vi "HEWH RLT PRAT.vi"() -> ()   [LabVIEW 2016] (continued)
        w1531 = 42 items=["No error", "Argument error", "Memory is full", "Out of zone", "End of file", "File already open", "Generic file I/O error", "File not found", "File permission error", "Disk is full", "Duplicate path", "Too many files open", "System feature not enabled", "Resource file not found", "Cannot add resource", "Resource not found", "Image not found", "Image memory error", "Pen does not exist", "Config type invalid", "Config token not found", "Config parse error", "Config memory error", "Bad external code format", "Bad external code offset", "External code not present", "Null window", "Destroy window error", "Null menu", "Print aborted", "Bad print record", "Print driver error", "Windows error during printing", "Memory error during printing", "Print dialog error", "Generic print error", "Invalid device refnum", "Device not found", "Device parameter error", "Device unit error", "Cannot open device", "Device call aborted", "Generic error", "Cancelled by user", "Object ID too low", "Object ID too high", "Object not in heap", "Unknown heap", "Unknown object (invalid DefProc)", "Unknown object (DefProc not in table)", "Message out of range", "Invalid (null) method", "Unknown message", "Manager call not supported", "Bad address", "Network operation in progress", "Network operation timed out", "Connection is busy", "Network attribute not supported", "Network error", "Address in use", "System out of memory", "Connection aborted", "Connection refused", "Not connected", "Already connected", "Connection closed", "Initialization error (interapplication manager)", "Bad occurrence", "Wait on unbound occurrence handler", "Occurrence queue overflow", "Datalog type conflict", "Unused", "Unrecognized type (interapplication manager)", "Memory corrupt", "Failed to make temporary DLL", "Old CIN version", "Drag socket not found", "Failed to load drop-object", "Failed to register OLE object", "Failed to release OLE object", "Format specifier type mismatch", "Unknown format specifier", "Too few format specifiers", "Too many format specifiers", "Scan failed", "Newer CIN version", "Error converting to variant", "Runtime menu error", "Password tampered", "Variant attribute not found", "Incompatible variant data type", "Event data is not available", "Event Store is not present", "Occurrence is not found", "Event Queue is not created", "Event info is not available", "Refnum passed is NULL", "Error retrieving Class GUID", "Error retrieving CoClass GUID", "Error retrieving TypeLib GUID.", "Bad built application magic bytes.", "Specific driver is different from the specific driver associated with the Logical Name.", "There is no session opened to the class driver.", "Max Error", "MAX - Error with config objects", "MAX - Error loading configuration", "MAX - Group not supported"]
        # "Current State"
        # "Handle mistyped state name (developer tool)"
        n704 = Format Into String(format string="Software Exception: Unhandled State \"%s\"." ("message"), error in=w1527, w1523) -> (resulting string=w1530:string, error out=w1529:errorcluster)  [unwired: 1 in]
        n705 = call <vilib>:"Error Cluster From Error Code.vi"("show call chain? (False)"=TRUE, "error in (no error)"=w1529, "error message (\"\")"=w1530, "error code (0)"=w1531) -> ("error out"=w1528:errorcluster)  [unwired: 5 in]
        n706 = call <vilib>:"Add State(s) to Queue__jki_lib_state_machine.vi"("State(s) in (\"\")"=w1526) -> ("States Out"=w1525:string)  [unwired: 14 in]
      }
      frame "Error Handler" {
        # "Unhandled Error -- Display it"
        # "Clear error"
        n707 = call <vilib>:"General Error Handler.vi"("error in (no error)"=w1534) -> ()  [unwired: 10 in, 5 out]
        n708 = call <vilib>:"Add State(s) to Queue__jki_lib_state_machine.vi"("State(s) in Front (\"\")"="/* Post Error States", "State(s) in (\"\")"=w1538) -> ("States Out"=w1537:string)  [unwired: 13 in]
      }
      frame "Exit" {
        n709 = flat-sequence {
          tunnel: w1543 -> [w1548]
          tunnel: [w1548] -> w1539
          tunnel: [w1551] -> w1541
          tunnel: w1539 -> [w1552]
          tunnel: [w1554] -> w1542
          tunnel: w1541 -> [w1554]
          tunnel: [TRUE] -> w1540
          frame #0 {
            n710 = local read "Start Draw"() -> (w1547:bool)
            n711 = case shown="True" w1547 {
              frame False {
              }
              frame True {
                n712 = while {
                  stop <- w1550 stop-if-true
                  n713 = local read "Draw Complete"() -> (w1550:bool)
                  n714 = Wait Until Next ms Multiple(millisecond multiple=u32 100) -> ()  [unwired: 1 out]
                }
              }
            }
          }
          frame #1 {
            n715 = call "HEWH RLT Release Notifier References.vi"("error in (no error)"=w1552) -> ("error out"=w1551:errorcluster)  [unwired: 10 in]
          }
          frame #2 {
          }
        }
        n716 = call <vilib>:"Add State(s) to Queue__jki_lib_state_machine.vi"("State(s) in (\"\")"=w1546) -> ("States Out"=w1545:string)  [unwired: 14 in]
        "DAQ Finished" <- w1540
      }
      frame "---------- Setup ----------" {
        n717 = call <vilib>:"Add State(s) to Queue__jki_lib_state_machine.vi"("State(s) in (\"\")"=w1558) -> ("States Out"=w1557:string)  [unwired: 14 in]
      }
      frame "Data: Initialize" {
        n718 = while {
          tunnel: ["Test Fixture Hardware"] -> w1570
          tunnel: [w1612] -> w1586
          tunnel: [w1611] -> w1585
          tunnel: [w1610] -> w1584
          tunnel: [w1609] -> w1583
          tunnel: [w1608] -> w1582
          tunnel: [w1607] -> w1581
          tunnel: ["Core HEWH Data Input A"] -> w1573
          tunnel: ["Core HEWH Data Input B"] -> w1580
          tunnel: ["Core HEWH Data Input C"] -> w1579
          tunnel: ["Core HEWH Data Input D"] -> w1578
          tunnel: ["File Locations A"] -> w1577
          tunnel: ["File Locations B"] -> w1576
          tunnel: ["File Locations C"] -> w1575
          tunnel: ["File Locations D"] -> w1574
          tunnel: [w1596] -> w1568
          tunnel: [w1595] -> w1567
          tunnel: [w1594] -> w1566
          tunnel: [w1593] -> w1565
          tunnel: [w1592] -> w1564
          tunnel: [w1591] -> w1563
          tunnel: [w1590] -> w1560
          tunnel: [w1589] -> w1559
          stop <- w1606 stop-if-true
          w1592 = dbl[][] []  # Plot Array C
          w1591 = dbl[][] []  # Plot Array D
          w1593 = dbl[][] []  # Plot Array B
          w1594 = dbl[][] []  # Plot Array A
          w1608 = string[][] []  # D Data Array
          w1609 = string[][] []  # C Data Array
          w1610 = string[][] []  # B Data Array
          w1611 = string[][] []  # A Data Array
          w1612 = string[][] []  # Save Data
          n719 = local read "Init Complete"() -> (w1606:bool)
          n720 = local read "LV Program"() -> (w1596:T24)
          n721 = Wait Until Next ms Multiple(millisecond multiple=u32 100) -> ()  [unwired: 1 out]
          n722 = local read "Analog Channel-List"() -> (w1589:string)
          n723 = local read "RLT Station Channels"() -> (w1607:T46)
          n724 = local read "Scan Rate (Seconds)"() -> (w1590:T10)
          n725 = local read "Power Analyzer"() -> (w1595:T11)
        }
        n726 = call <vilib>:"Add State(s) to Queue__jki_lib_state_machine.vi"("State(s) in (\"\")"=w1588) -> ("States Out"=w1587:string)  [unwired: 14 in]
        n727 = Bundle("Test Fixture Hardware"=w1570, "Save Data"=w1586, "A Data Array"=w1585, "B Data Array"=w1584, "C Data Array"=w1583, "D Data Array"=w1582, "RLT Station Channels"=w1581, "Core HEWH Data Input A"=w1573, "Core HEWH Data Input B"=w1580, "Core HEWH Data Input C"=w1579, "Core HEWH Data Input D"=w1578, "File Locations A"=w1577, "File Locations B"=w1576, "File Locations C"=w1575, "File Locations D"=w1574, "Plot Array A"=w1566, "Plot Array B"=w1565, "Plot Array C"=w1564, "Plot Array D"=w1563, "Scan Rate (Seconds)"=w1560) -> (w1571:T80)  [unwired: 1 in]
        n728 = Unbundle By Name(w1570) -> ("Analog Data.Yokogawa.MW100"=→"MW100":refnum<visa-resource-name>, "Power.Yokogawa.WT210.Power VISA Yokogawa WT210"=→"Yokogawa WT210":refnum<visa-resource-name>)
        n729 = Bundle By Name(cluster=w1571, "Core HEWH Data Input A.HEWH Specific DAQ.Power Analyzer"=w1567, "Core HEWH Data Input B.HEWH Specific DAQ.Power Analyzer"=w1567, "Core HEWH Data Input C.HEWH Specific DAQ.Power Analyzer"=w1567, "Core HEWH Data Input D.HEWH Specific DAQ.Power Analyzer"=w1567, "Core HEWH Data Input A.LV Program"=w1568, "Core HEWH Data Input B.LV Program"=w1568, "Core HEWH Data Input C.LV Program"=w1568, "Core HEWH Data Input D.LV Program"=w1568, "Test Fixture Hardware.Analog Data.Agilent.TC Channels-List"=w1559) -> (w1572:T80)
      }
      frame "Initialize Equipment" {
        w1624 = 0 ("Core HEWH Data Input A.Draw Count")
        # "The Initialize Equipment only requires VISA connections. We use\na single MW100, WT Series, and 34972A"
        n730 = Unbundle By Name(w1632) -> ("Test Fixture Hardware"=w1633:T47, "Core HEWH Data Input A"=w1634:T12, "Test Fixture Hardware.Gas Meter COM Ports.Gas Meter 1"=w1619:refnum<visa-resource-name>)
        n731 = local read "Use Agilent?"() -> (w1623:bool)
        n732 = call "HEWH Initialize Equipmet.vi"("Refnum in"=w1625, "Use Agilent?"=w1623, "Error In"=w1626, "Pressurize Tank"="Pressurize Tank?", "Core HEWH Data"=w1634, "Test Fixture Hardware"=w1633) -> ("Error Out"=w1621:errorcluster)  [unwired: 4 in, 1 out]
        n733 = call "FMA1600A General Setup.vi"("baud rate (19200)"=u32 19200 ("baud rate (9600)"), "Unit ID"="A", "error in (no error)"=w1621, "Set STP Register"=FALSE, "VISA Refnum in"=w1619) -> ("error out"=w1617:errorcluster, "VISA Refnum out"=w1614:refnum<visa-resource-name>)  [unwired: 4 in, 1 out]
        n734 = call <vilib>:"Add State(s) to Queue__jki_lib_state_machine.vi"("State(s) in (\"\")"=w1637) -> ("States Out"=w1636:string)  [unwired: 14 in]
        n735 = Bundle By Name(cluster=w1632, "Core HEWH Data Input A.Station ID"=Station_ID_Selector."A", "Core HEWH Data Input B.Station ID"=Station_ID_Selector."B", "Core HEWH Data Input C.Station ID"=Station_ID_Selector."C", "Core HEWH Data Input D.Station ID"=Station_ID_Selector."D", "Core HEWH Data Input A.Draw Count"=w1624, "Core HEWH Data Input B.Draw Count"=w1624, "Core HEWH Data Input C.Draw Count"=w1624, "Core HEWH Data Input D.Draw Count"=w1624, "Test Fixture Hardware.Gas Meter COM Ports.Gas Meter 1"=w1614) -> (w1631:T80)
        n736 = call <vilib>:"Clear Errors.vi"("error in (no error)"=w1617, "specific error code to clear (0: all)"=0) -> ("error out"=w1616:errorcluster)  [unwired: 4 in, 1 out]
      }
      frame "Get Software Version A" {
        w1645 = "." ("string")
        w1652 = GEA2_Commands."RQST_Software_Version" ("GEA2 Commands and Requests")
        n737 = Unbundle By Name(w1643) -> ("Board ID"=→"Board ID A":string, "GEA2 Reference Out"=w1642:refnum<k24>, "GEA2 Event Registration"=w1641:refnum<event-registration>)
        n738 = call "HEWH_DSM_CMD.vi"("GEA2 Commands and Requests"=w1652) -> ("Input Data"=w1651:T74)  [unwired: 8 in, 1 out]
        n739 = call "GEA2 Send and Receive Message.vi"("GEA2 Reference In"=w1642, "Input Data"=w1651, "GEA2 Event Registration"=w1641, "Error In"=w1640) -> ("Converted Data Out"=w1653:T81, "Error Out"=w1639:errorcluster)  [unwired: 6 in, 4 out]
        n740 = call "GEA2 Message Decoder.vi"("GEA2 Commands and Requests"=w1652, "Coverted Data Out"=w1653) -> ("GEA Information Out"=w1650:T57)  [unwired: 9 in]
        n741 = Unbundle By Name(w1650) -> ("Software Version.Critical Major SW Version"=w1649:string, "Software Version.Critical Minor SW Version"=w1648:string, "Software Version.Major SW Version"=w1647:string, "Software Version.Minor SW Version"=w1646:string)
        n742 = Concatenate Strings(w1649, w1645, w1648, w1645, w1647, w1645, w1646) -> (→"Software Version A":string)
        n743 = call <vilib>:"Add State(s) to Queue__jki_lib_state_machine.vi"("State(s) in (\"\")"=w1656) -> ("States Out"=w1655:string)  [unwired: 14 in]
      }
      frame "Get Software Version B" {
        w1664 = "." ("string")
        w1671 = GEA2_Commands."RQST_Software_Version" ("GEA2 Commands and Requests")
        n744 = Unbundle By Name(w1662) -> ("Board ID"=→"Board ID B":string, "GEA2 Reference Out"=w1661:refnum<k24>, "GEA2 Event Registration"=w1660:refnum<event-registration>)
        n745 = call "HEWH_DSM_CMD.vi"("GEA2 Commands and Requests"=w1671) -> ("Input Data"=w1670:T74)  [unwired: 8 in, 1 out]
        n746 = call "GEA2 Send and Receive Message.vi"("GEA2 Reference In"=w1661, "Input Data"=w1670, "GEA2 Event Registration"=w1660, "Error In"=w1659) -> ("Converted Data Out"=w1672:T81, "Error Out"=w1658:errorcluster)  [unwired: 6 in, 4 out]
        n747 = call "GEA2 Message Decoder.vi"("GEA2 Commands and Requests"=w1671, "Coverted Data Out"=w1672) -> ("GEA Information Out"=w1669:T57)  [unwired: 9 in]
        n748 = Unbundle By Name(w1669) -> ("Software Version.Critical Major SW Version"=w1668:string, "Software Version.Critical Minor SW Version"=w1667:string, "Software Version.Major SW Version"=w1666:string, "Software Version.Minor SW Version"=w1665:string)
        n749 = Concatenate Strings(w1668, w1664, w1667, w1664, w1666, w1664, w1665) -> (→"Software Version B":string)
        n750 = call <vilib>:"Add State(s) to Queue__jki_lib_state_machine.vi"("State(s) in (\"\")"=w1675) -> ("States Out"=w1674:string)  [unwired: 14 in]
      }
      frame "Get Software Version C" {
        w1683 = "." ("string")
        w1690 = GEA2_Commands."RQST_Software_Version" ("GEA2 Commands and Requests")
        n751 = Unbundle By Name(w1681) -> ("Board ID"=→"Board ID C":string, "GEA2 Reference Out"=w1680:refnum<k24>, "GEA2 Event Registration"=w1679:refnum<event-registration>)
        n752 = call "HEWH_DSM_CMD.vi"("GEA2 Commands and Requests"=w1690) -> ("Input Data"=w1689:T74)  [unwired: 8 in, 1 out]
        n753 = call "GEA2 Send and Receive Message.vi"("GEA2 Reference In"=w1680, "Input Data"=w1689, "GEA2 Event Registration"=w1679, "Error In"=w1678) -> ("Converted Data Out"=w1691:T81, "Error Out"=w1677:errorcluster)  [unwired: 6 in, 4 out]
        n754 = call "GEA2 Message Decoder.vi"("GEA2 Commands and Requests"=w1690, "Coverted Data Out"=w1691) -> ("GEA Information Out"=w1688:T57)  [unwired: 9 in]
        n755 = Unbundle By Name(w1688) -> ("Software Version.Critical Major SW Version"=w1687:string, "Software Version.Critical Minor SW Version"=w1686:string, "Software Version.Major SW Version"=w1685:string, "Software Version.Minor SW Version"=w1684:string)
        n756 = Concatenate Strings(w1687, w1683, w1686, w1683, w1685, w1683, w1684) -> (→"Software Version C":string)
        n757 = call <vilib>:"Add State(s) to Queue__jki_lib_state_machine.vi"("State(s) in (\"\")"=w1694) -> ("States Out"=w1693:string)  [unwired: 14 in]
      }
      frame "Get Software Version D" {
        w1702 = "." ("string")
        w1709 = GEA2_Commands."RQST_Software_Version" ("GEA2 Commands and Requests")
        n758 = Unbundle By Name(w1700) -> ("Board ID"=→"Board ID D":string, "GEA2 Reference Out"=w1699:refnum<k24>, "GEA2 Event Registration"=w1698:refnum<event-registration>)
        n759 = call "HEWH_DSM_CMD.vi"("GEA2 Commands and Requests"=w1709) -> ("Input Data"=w1708:T74)  [unwired: 8 in, 1 out]
        n760 = call "GEA2 Send and Receive Message.vi"("GEA2 Reference In"=w1699, "Input Data"=w1708, "GEA2 Event Registration"=w1698, "Error In"=w1697) -> ("Converted Data Out"=w1710:T81, "Error Out"=w1696:errorcluster)  [unwired: 6 in, 4 out]
        n761 = call "GEA2 Message Decoder.vi"("GEA2 Commands and Requests"=w1709, "Coverted Data Out"=w1710) -> ("GEA Information Out"=w1707:T57)  [unwired: 9 in]
        n762 = Unbundle By Name(w1707) -> ("Software Version.Critical Major SW Version"=w1706:string, "Software Version.Critical Minor SW Version"=w1705:string, "Software Version.Major SW Version"=w1704:string, "Software Version.Minor SW Version"=w1703:string)
        n763 = Concatenate Strings(w1706, w1702, w1705, w1702, w1704, w1702, w1703) -> (→"Software Version D":string)
        n764 = call <vilib>:"Add State(s) to Queue__jki_lib_state_machine.vi"("State(s) in (\"\")"=w1713) -> ("States Out"=w1712:string)  [unwired: 14 in]
      }
      frame "Update File Locations" {
        n765 = flat-sequence {
          tunnel: w1715 -> [w1729]
          tunnel: w1720 -> [w1728]
          tunnel: w1719 -> [w1727]
          tunnel: w1718 -> [w1726]
          tunnel: w1717 -> [w1725]
          tunnel: [w1724] -> w1716
          tunnel: w1716 -> [w1731]
          tunnel: [w1731] -> w1714
          frame #0 {
            n766 = Bundle By Name(cluster=w1729, "File Locations A"=w1728, "File Locations B"=w1727, "File Locations C"=w1726, "File Locations D"=w1725) -> (w1724:T80)
          }
          frame #1 {
            n767 = Unbundle By Name(w1731) -> ("Core HEWH Data Input A"=w1735:T12, "Core HEWH Data Input B"=w1734:T12, "Core HEWH Data Input C"=w1733:T12, "Core HEWH Data Input D"=w1732:T12, "Scan Rate (Seconds)"=→"Scan Rate (Default)":T10)
            n768 = local write "Core HEWH Data Input A"(w1735) -> ()
            n769 = local write "Core HEWH Data Input B"(w1734) -> ()
            n770 = local write "Core HEWH Data Input C"(w1733) -> ()
            n771 = local write "Core HEWH Data Input D"(w1732) -> ()
          }
          frame #2 {
            "Start Draw Loop" <- TRUE ("Init Complete")
          }
        }
        n772 = call <vilib>:"Add State(s) to Queue__jki_lib_state_machine.vi"("State(s) in (\"\")"=w1723) -> ("States Out"=w1722:string)  [unwired: 14 in]
      }
      frame "Load Configuration" {
        n773 = Unbundle By Name(w1742) -> ("Core HEWH Data Input A.LV Program"=w1746:T24, "File Locations A"=w1745:T2)
        n774 = call "Save File DOE File Setup.vi"("Filepath In"=w1745, "Washer Controls In"=T75 {"Test Fixture Hardware"={"Power "={"Yokogawa"={"WT210"={"Sample Rate (1: 0.25s)"=1, "A Range (12: 20A)"=12, "V Range (6: 600V)"=4, "Power VISA Yokogawa WT210"="WT210"}, "WT500"={"Power VISA Yokogawa WT500"="WT500", "V Range (8: 1000V)"=0, "I Range (7: 40A)"=0, "Update Rate (3: 500ms)"=2}, "WT310_2"={"Sample Rate (1: 0.25s)"=1, "A Range (12: 20A)"=11, "V Range (6: 600V)"=4, "Power VISA Yokogawa WT310_2"=""}, "WT310_3"={"Sample Rate (1: 0.25s)"=1, "A Range (12: 20A)"=11, "V Range (6: 600V)"=4, "Power VISA Yokogawa WT310_3"=""}}, "Aplus"={"Aplus IP Address"="192.168.1.101", "Remote Port"=502, "Instrument"="APLUS", "Instr Driver Revision"="1.03.0053"}, "Power Limits"={"Crest Factor"={"Upper Limit"=1.49, "Lower Limit"=1.34}, "Harmonic Content"={"Uthd"=2.0}, "Voltage"={"% Error"=2.0}, "Stability"={"<1 Watt "={"Wattage"=1.0, "Slope (mW/H)"=10.0}, ">1 Watt"={"1%Power/Hour"=1.0}}}, "Nominal Voltage"=120, "Time Limit (s)"=10800.0, "Power Variation Limit (%)"=50.0, "Power Supply"={"Chroma 61605"="CHROMA", "Use Chroma?"=FALSE}}, "Weight Scale"={"Com Options"={"IND560Scale VISA"="IND560", "IP Address"="192.168.1.50", "Remote Port"=502, "Setra Scale VISA"="COM3", "GSE 350"="GSE350"}, "Select Scale"=""}, "Flow Rates"={"Laurel Cold IP Address"="", "Laurel Hot IP Address"="34972A_2", "Hot Water Laurel VISA"="LaurelMeter_Hot", "Cold Water Laurel VISA"="LaurelMeter_Cold", "Remote Port"=0, "Laurel Communication Type"="", "Meters To Collect (Hot Cold)"="", "HOT Laurel Reference"=refnum, "COLD Laurel Reference"=refnum}, "Analog Data"={"Agilent"={"Agilent 34972_1"="34972A_1", "Agilent 34972_2"="34972A_2", "Agilent 34972_3"="34972A_3", "Agilent 34972_4"="34972A_4", "Agilent 34972_5"="34972A_5", "Agilent 34972_6"="34972A_6", "Agilent Gain"=0.0, "TC Type (K,J,T)"="", "Instrument IDN?"="", "TC Channels-List"="", "Analog Channels-List"="", "Agilent Cluster Array"=[], "TC Channels-List 2"="", "Analog Channels-List 2"=""}, "Yokogawa"={"MW100"="MW100", "Intellifaucet"=FALSE}, "Select Analog"="", "TC Coefficients"={"TC Coefficients 1"=[], "TC Coefficients 2"=[], "TC Coefficients 3"=[], "TC Coefficients 4"=[], "TC Coefficients 5"=[], "TC Coefficients 6"=[], "TC Coefficients 7"=[]}, "NI Tasks (Dryer DOE)"=["TC Temps-Module 1", "TC Temps-Module 2", "TC Temps-Module 3", "TC Temps-Module 4", "TC Temps-Module 5", "Gas and Temp-Module 6", "AC_DC Events-Module 7"], "Laurel Analog"={"Laurel IP (Water Temp)"="", "Laurel IP (Pressure)"=""}}, "ITHX-Temp Humidity"={"IP Address 1"="", "Remote Port"=0, "IP Address 2"="", "IP Address 3"=""}, "Gas Meter COM Ports"={"Gas Meter 1"="COM3", "Gas Meter 2"="COM4", "Gas Meter 3"="COM5", "Gas Meter 4"="COM6", "Gas Meter 5"="COM7", "Gas Meter 6"="COM8"}, "Barometric Pressure"={"HEISE 901A"="HEISE", "Use Barometer?"=FALSE}}, "GEA2"={"Address"=35, "Source"=228, "Viper/Hawk"=0}, "DOE Capacity Measurments"={"Weight 1"=35.0, "Model Number 1"="", "Temp 1"=0.0, "Serial Number 1"="", "Lab Number 1"="", "Lab Number 2"="", "Serial Number 2"="", "Temp 2"=0.0, "Model Number 2"="", "Weight 2"=0.0, "Lab Number 3"="", "Serial Number 3"="", "Temp 3"=0.0, "Model Number 3"="", "Weight 3"=0.0, "Lab Number 4"="", "Serial Number 4"="", "Temp 4"=0.0, "Model Number 4"="", "Weight 4"=0.0, "Capacity Measurment Output String"=[]}, "Initialize.Washer In"={"Appliance Details"={"FileVersionInfo"={"FileVersion"="", "ProductName"="", "InternalName"="", "CompanyName"="", "LegalCopyright"="", "FileDescription"=""}, "Dishwasher Info"={"Open Cup Weight (gm):"=0.0, "Auto Cup Weight (gm):"=0.0, "Detergent-Dish:"="", "Inlet Temperature-Dish:"="", "Cycle Mode-Dish:"="", "Unit Control-Dish:"="", "Manufacturer-Dish:"=""}, "Washer Info"={"Hot Water Temperature (Fahrenheit):"="", "Cold Water Temperature (Fahrenheit):"="", "Capacity (cu.ft):"=0.0, "Initial Cloth Weight:"=0.0, "Cloth Lot:"=60, "Model Family:"="", "Program Name:"="", "Cycle Selection:"="", "Wash Temperature:"="", "Rinse Temperature:"="", "Load Size:"=""}, "File Name Output Array"=[], "Calibration Output Array"=[], "Appliance Common"={"Engineer:"="", "Model Number:"="", "Serial Number:"="", "Comments:"="", "Station ID:"="", "Technician:"="", "TR Number:"="", "Lab ID:"="", "Voltage:"="", "Water Pressure (PSI):"="", "Test Date:"="", "Computer Name:"="", "IP Address:"="", "Ambient RH:"="", "Frequency:"="", "Build:"="", "Filename:"="", "Test Type:"="", "Load Run #:"=17, "Ambient Temperature (F):"="", "File Path:"=path "", "Cycles Per Year"=0}, "Water Heater"={"Heating Mode:"=""}, "Dryer"={"Heat Setting:"="", "Washer Water Temperature (60 ± 5°F):"=7, "Water Hardness (PPM):"=7, "Dryness Setting:"="", "Dryer Type:"="", "Exhaust:"="", "Drying Cycle:"="", "Load Type:"="", "Nominal Load Weight"="", "Dryer Initial IMC Data"={"Measured IMC (lbs)"=100.0, "Actual Initial RMC (%)"=7.0, "RMC (Desired %)"=5.0, "Bone Dry Wt(lbs)"=60.0, "Tolerance(%)"=0.0, "Actual Final RMC (%)"=0.0, "CEF (lbf/kWh)"=0.0, "Minimum Weight (lbf)"=0.0, "Average Weight (lbf)"=0.0, "Maximum Weight (lbf)"=0.0, "Measured IMC In Range?"=FALSE, "Moisture Reduction Factor"=55.5, "Field Use Factor"=1.04, "Empty Dryer Cold Weigth"=0.0, "Energy Standard"=enum."D2-Automatic Dryer", "Weight Cloth (lbs)"=0.0, "Relative Moisture Content (%)"=0.0, "Relative Moisture Content - Avg (%)"=0.0}}}, "Display Data (RLT)"={"Status Color"=0, "Serial Number Display"="", "Cycle Count Display"=0, "Station Label Display"="", "Current Run Start Time Display"=0.0, "Board ID Display"="", "RPM Display"=0, "Current Display"=0.0, "Current Path Display"=path "", "Saving Display"=FALSE, "Unit Type Display"=enum."", "Total Time On Display"=0.0, "UI Button"=FALSE}}}, "error in (no error)"=w1748, "Config State"=Save_File_DOE_Configuration_State."Load Config", "LV Program"=w1746) -> ("Washer Controls Out"=w1743:T75, "Filepath Out"=w1738:T2, "error out"=w1747:errorcluster)  [unwired: 12 in]
        n775 = Unbundle By Name(w1743) -> ("Test Fixture Hardware.ITHX-Temp Humidity.IP Address 1"=w1741:string, "Test Fixture Hardware.Flow Rates.Laurel Hot IP Address"=w1739:string)
        "ITHX-Temp Humidity" <- w1741
        "Laurel Hot IP Address" <- w1739
        n776 = call <vilib>:"Add State(s) to Queue__jki_lib_state_machine.vi"("State(s) in (\"\")"=w1751) -> ("States Out"=w1750:string)  [unwired: 14 in]
        n777 = Bundle By Name(cluster=w1742, "Test Fixture Hardware.ITHX-Temp Humidity.Remote Port"=u16 2000, "Test Fixture Hardware.ITHX-Temp Humidity.IP Address 1"=w1741, "Test Fixture Hardware.Flow Rates.Laurel Hot IP Address"=w1739, "File Locations A"=w1738, "File Locations B"=w1738, "File Locations C"=w1738, "File Locations D"=w1738) -> (w1737:T80)
      }
      frame "Init Hot Laurel" {
        n778 = Unbundle By Name(w1755) -> ("Test Fixture Hardware.Flow Rates.Laurel Hot IP Address"=w1752:string)
        n779 = Equal?(x=w1752, y="") -> (x = y?=w1753:bool)
        n780 = case shown="False" w1753 {
          tunnel: w1752 -> [_ w1763]
          tunnel: w1757 -> [w1760 w1762]
          tunnel: [w1760 w1765] -> w1756
          frame True {
          }
          frame False {
            n781 = call "Emerson 5700 Basic Tester.vi"("Error In"=w1762, "Remote IP Address"=w1763) -> ("Error Out"=w1761:errorcluster)  [unwired: 8 in, 1 out]
            n782 = case shown="Error" w1761 {
              selector: w1761 -> [w1774 _]
              tunnel: [w1769 w1781] -> w1765
              tunnel: w1763 -> [w1767 w1779]
              tunnel: [TRUE ("Use Emerson 5700") FALSE ("Use Emerson 5700")] -> w1764
              frame No Error {
                w1768 = T82 4 items=["Start/Stop Inventory 1"=367, "Start/Stop Inventory 2"=368, "Start/Stop all Totalizers and Inventories"=2, "Reset all Totalizers"=3, "Reset all Inventories"=4, "Reset Totalizer 1"=56, "Reset Totalizer 2"=57] ("Reset all Totalizers. 2")
                w1772 = T82 3 items=["Start/Stop Inventory 1"=367, "Start/Stop Inventory 2"=368, "Start/Stop all Totalizers and Inventories"=2, "Reset all Totalizers"=3, "Reset all Inventories"=4, "Reset Totalizer 1"=56, "Reset Totalizer 2"=57] ("Reset all Totalizers. 2")
                n783 = property on="Reset Inventory" class="Bool"("DisabledEnum"=T67."Enabled" ("Disabled")) -> ()  [unwired: 2 in, 2 out]
                n784 = call "Emerson 5700 Reset Totalizers.vi"("Reset all Totalizers. 2"=w1772, "Error In"=w1774, "Coil"=TRUE, "address"=w1767) -> ("Error Out"=w1770:errorcluster)  [unwired: 7 in]
                n785 = call "Emerson 5700 Reset Totalizers.vi"("Reset all Totalizers. 2"=w1768, "Error In"=w1770, "Coil"=TRUE, "address"=w1767) -> ("Error Out"=w1769:errorcluster)  [unwired: 7 in]
              }
              frame Error {
                n786 = for {
                  N: 2 -> [_]
                  tunnel: w1779 -> [w1785]
                  tunnel: errorcluster {"status"=FALSE, "code"=0, "source"=""} ("Error Out") -> [w1784]
                  tunnel: [w1783] -> w1781
                  n787 = First Call?() -> (First Call?: T/F=w1787:bool)
                  n788 = call "Laurel Data GET Top Level.vi"("Laurel IP Address"=w1785, "Laurel Serial Commands"=T79 "*1C1", "First Call?"=w1787, "error in (no error)"=w1784, "Laurel Communication Type"="TCP") -> ("error out"=w1783:errorcluster)  [unwired: 5 in, 5 out]
                }
                n789 = property on="Reset Inventory" class="Bool"("DisabledEnum"=T67."Disabled and Grayed Out" ("Disabled")) -> ()  [unwired: 2 in, 2 out]
              }
            }
            "Use Emerson 5700" <- w1764
          }
        }
        n790 = call <vilib>:"Add State(s) to Queue__jki_lib_state_machine.vi"("State(s) in (\"\")"=w1759) -> ("States Out"=w1758:string)  [unwired: 14 in]
      }
      frame "Shutdown Equipment" {
        n791 = Unbundle By Name(w1797) -> ("Test Fixture Hardware"=w1796:T47, "Core HEWH Data Input A"=w1795:T12, "Test Fixture Hardware.Gas Meter COM Ports.Gas Meter 1"=w1789:refnum<visa-resource-name>)
        n792 = local read "Pressurize Tank?"() -> (w1794:bool)
        n793 = local read "Get Gas Data"() -> (w1788:bool)
        n794 = call "HEWH Close Equipmet.vi"("Refnum in"=w1792, "Pressurize Tank"=w1794, "Error In"=w1793, "Core HEWH Data"=w1795, "Test Fixture Hardware In"=w1796) -> ("Error Out"=w1791:errorcluster)  [unwired: 5 in, 1 out]
        n795 = case shown="True" w1788 {
          tunnel: w1791 -> [w1800 w1803]
          tunnel: [w1800 w1802] -> w1790
          tunnel: w1789 -> [_ w1801]
          frame False {
          }
          frame True {
            n796 = call "FMA1600A Close.vi"("error in (no error)"=w1803, "VISA Refnum in"=w1801) -> ("error out"=w1802:errorcluster)  [unwired: 9 in]
          }
        }
        n797 = call <vilib>:"Add State(s) to Queue__jki_lib_state_machine.vi"("State(s) in (\"\")"=w1799) -> ("States Out"=w1798:string)  [unwired: 14 in]
      }
      frame "---------- Data ----------" {
        n798 = call <vilib>:"Add State(s) to Queue__jki_lib_state_machine.vi"("State(s) in (\"\")"=w1807) -> ("States Out"=w1806:string)  [unwired: 14 in]
      }
      frame "Data: Get Time" {
        w1808 = i16 2 ("precision (6)")
        w1809 = TRUE ("Add Software Elapsed Time")
        w1835 = string[][] [] ("A Data Array")
        # "allows reset after purge"
        # "Reset Array"
        n799 = call "UTILITY Elapsed Time.vi"("error in (no error)"=w1812, "Reset Timer"="Reset Timer (Main)") -> ("error out"=w1811:errorcluster, "Main Loop Rate"=→"DAQ Loop Rate":dbl, "Elapsed Time"=w1810:dbl)  [unwired: 5 in, 2 out]
        "Software Elapsed Time" <- w1810
        n800 = Bundle By Name(cluster=w1833, "A Data Array"=w1835, "B Data Array"=w1835, "C Data Array"=w1835, "D Data Array"=w1835) -> (w1834:T80)
        n801 = local read "A Timer"() -> (w1824:dbl)
        n802 = local read "B Timer"() -> (w1820:dbl)
        n803 = call "UTILITY Elapsed Time General Info.vi"("precision (6)"=w1808, "Add Software Elapsed Time"=w1809, "Error In"=w1811, "Software Elapsed Time"=w1810, "Elapsed Time (sec)"=w1824) -> ("Error Out"=w1822:errorcluster, "Total Array"=w1823:string[][])  [unwired: 2 in, 3 out]
        n804 = local read "C Timer"() -> (w1815:dbl)
        n805 = call "UTILITY Elapsed Time General Info.vi"("precision (6)"=w1808, "Add Software Elapsed Time"=w1809, "Error In"=w1822, "Software Elapsed Time"=w1810, "Elapsed Time (sec)"=w1820) -> ("Error Out"=w1819:errorcluster, "Total Array"=w1821:string[][])  [unwired: 2 in, 3 out]
        n806 = call "UTILITY Elapsed Time General Info.vi"("precision (6)"=w1808, "Add Software Elapsed Time"=w1809, "Error In"=w1819, "Software Elapsed Time"=w1810, "Elapsed Time (sec)"=w1815) -> ("Error Out"=w1818:errorcluster, "Total Array"=w1817:string[][])  [unwired: 2 in, 3 out]
        n807 = local read "D Timer"() -> (w1814:dbl)
        n808 = call "UTILITY Elapsed Time General Info.vi"("precision (6)"=w1808, "Add Software Elapsed Time"=w1809, "Error In"=w1818, "Software Elapsed Time"=w1810, "Elapsed Time (sec)"=w1814) -> ("Error Out"=w1813:errorcluster, "Total Array"=w1816:string[][])  [unwired: 2 in, 3 out]
        n809 = case shown="\"Single Station\", Default" w1829 {
          tunnel: w1816 -> [_ w1844]
          tunnel: w1817 -> [_ w1843]
          tunnel: w1821 -> [_ w1842]
          tunnel: w1823 -> [w1840 w1841]
          tunnel: [w1839 w1844] -> w1825
          tunnel: [w1839 w1843] -> w1826
          tunnel: [w1839 w1842] -> w1827
          tunnel: [w1840 w1841] -> w1828
          frame "Single Station", Default {
            w1839 = string[][] [] ("Total Array")
          }
          frame "Four Stations" {
          }
        }
        n810 = call <vilib>:"Add State(s) to Queue__jki_lib_state_machine.vi"("State(s) in (\"\")"=w1838) -> ("States Out"=w1837:string)  [unwired: 14 in]
        n811 = flat-sequence {
          tunnel: w1813 -> [w1846]
          tunnel: [w1846] -> w1831
          frame #0 {
            w1845 = FALSE ("Reset Timer")
            n812 = local write "Reset Timer (Main)"(w1845) -> ()
            n813 = local write "Reset Timer (A)"(w1845) -> ()
            n814 = local write "Reset Timer (B)"(w1845) -> ()
            n815 = local write "Reset Timer (C)"(w1845) -> ()
            n816 = local write "Reset Timer (D)"(w1845) -> ()
          }
        }
        n817 = Bundle By Name(cluster=w1834, "A Data Array"=w1828, "B Data Array"=w1827, "C Data Array"=w1826, "D Data Array"=w1825) -> (w1836:T80)
      }
      frame "Data: Get MW100 (Station A)" {
        w1851 = "A" ("Prat Station")
        n818 = Unbundle By Name(w1878) -> ("A Data Array"=w1880:string[][], "Test Fixture Hardware"=w1871:T47, "Core HEWH Data Input A"=w1870:T12, "Test Fixture Hardware.Power.Yokogawa.WT210.Power VISA Yokogawa WT210"=w1863:refnum<visa-resource-name>, "RLT Station Channels.MW100.Station A Channels, MW100"=w1866:string[][])
        n819 = property on="Cycle Count Display" class="DigNum (strict)"() -> ("Value"=w1852:i32)  [unwired: 2 in, 2 out]
        n820 = local read "Use Emerson 5700"() -> (w1847:bool)
        n821 = Unbundle By Name(w1871) -> ("Flow Rates.Laurel Hot IP Address"=w1853:string, "Analog Data.Yokogawa.MW100"=w1875:refnum<visa-resource-name>)
        n822 = call "UTILITY Aquire Semaphore.vi"("error in (no error)"=w1874, "Refnum in"=w1873) -> ("error out"=w1876:errorcluster, "Refnum out"=w1877:T56)  [unwired: 7 in, 1 out]
